vi "Get Process Control Actions.vi"(8 "error in (no error)":errorcluster {"code" format="Error %.0f"}, 11 "VIDoc Printer In":refnum<class "VIDoc Printer.lvclass">) -> (0 "error out":errorcluster {"code" format="Error %.0f"}, 2 "Process Control Actions":T1[](array[typedef]), 3 "VIDoc Printer Out":refnum<class "VIDoc Printer.lvclass">)   [LabVIEW 2023, in "VIDoc Printer.lvlib" / "VIDoc Printer.lvclass"]
uses:
  VIDoc Printer.lvclass
  VIDoc Printer.lvclass/VIDoc Printer.ctl
  Controls/Process Control Enum.ctl
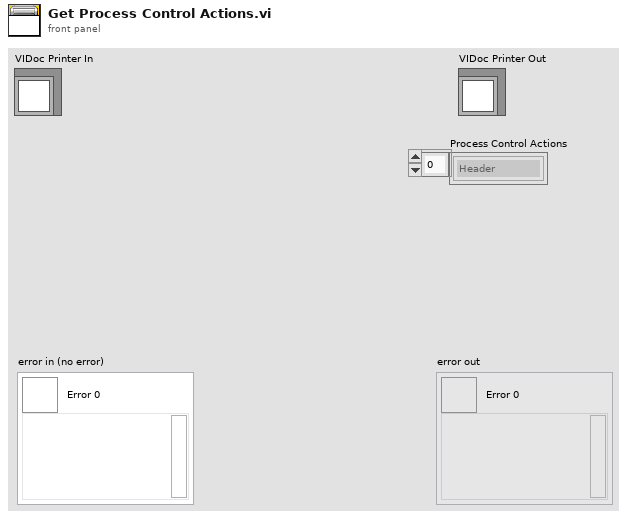
[diagram p1: front panel]
types:
  T1 = typedef "VIDoc Printer.lvlib/VIDoc Printer.lvclass/Process Control Enum.ctl" = enum16{"Header", "Memory", "By Folder", "By Tree", "By List", "Controls"}
  T2 = typedef "VIDoc Printer.lvlib/Printer Settings.lvclass/Detail Level Enum.ctl" = enum16{"None", "Minimal", "Standard", "Full"}
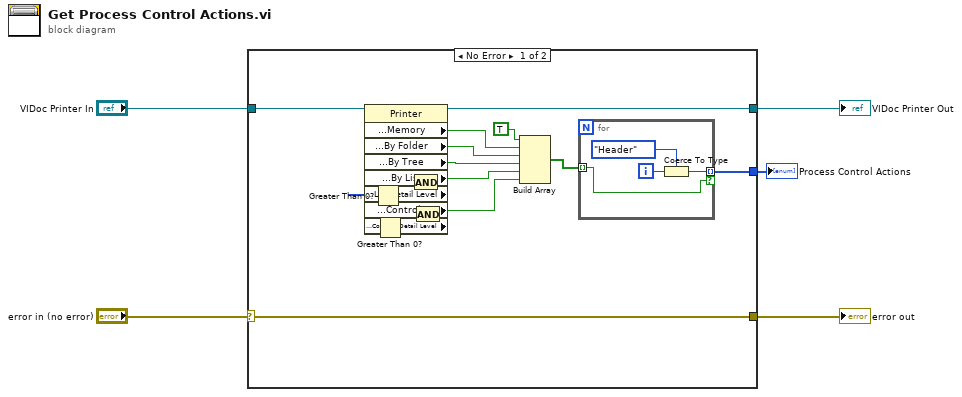
[diagram p0: block diagram]
diagram:
  n1 = case shown="No Error" "error in (no error)" {
    selector: "error in (no error)" -> [w22 w28]
    tunnel: [w22 w28] -> w4
    tunnel: [w14 w27] -> w2
    tunnel: "VIDoc Printer In" -> [w15 w27]
    tunnel: [w12 _] -> w1
    frame No Error {
      n2 = property class="Printer"(reference=w15) -> (reference out=w14:refnum<class "VIDoc Printer.lvclass">, "Properties:Settings:Control Members:Memory"=w20:bool, "Properties:Settings:Control Members:By Folder"=w19:bool, "Properties:Settings:Control Members:By Tree"=w18:bool, "Properties:Settings:Control Members:By List"=w17:bool, "Properties:Settings:Control Members:List Detail Level"=w10:T2, "Properties:Settings:Control Members:Controls"=w16:bool, "Properties:Settings:Control Members:Controls Detail Level"=w11:T2)  [unwired: 1 in, 1 out]
      n3 = Greater Than 0?(x=w10) -> (x > 0?=w8:bool)
      n4 = Greater Than 0?(x=w11) -> (x > 0?=w6:bool)
      n5 = And(x=w17, y=w8) -> (x .and. y?=w9:bool)
      n6 = And(x=w16, y=w6) -> (x .and. y?=w7:bool)
      n7 = Build Array(TRUE ("element"), w20, w19, w18, w9, w7) -> (w13:bool[])
      n8 = for {
        tunnel: w13 -> [w23] mode=indexing
        tunnel: [w24] -> w12 mode=indexing if=w23
        i -> [w25]
        n9 = Coerce To Type(0:w25, 1:Process_Control_Enum."Header") -> (2:w24:T1)
      }
    }
    frame Error {
    }
  }
  "error out" <- w4
  "VIDoc Printer Out" <- w2
  "Process Control Actions" <- w1
